vi "ABR-Set Level.vi"(0 "Runtime":T1, 11 "error in (no error)":errorcluster) -> (4 "Runtime out":T1, 14 "Level":dbl, 15 "error out":errorcluster)   [LabVIEW 2020]
uses:
  TypeDefs/ABR-Runtime Data.ctl
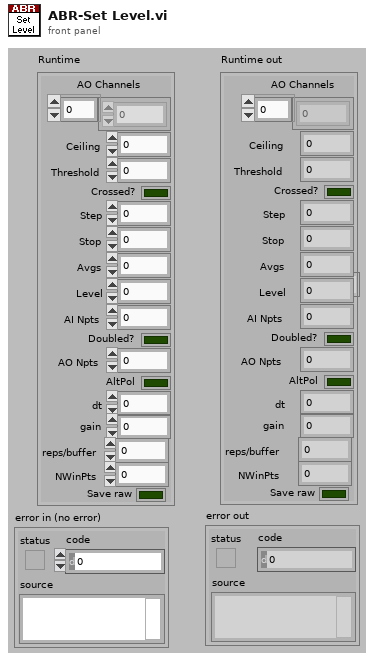
[diagram p1: front panel]
types:
  T1 = typedef "ABR-Runtime Data.ctl" = cluster{"AO Channels":i32[], "Ceiling":dbl, "Threshold":dbl, "Crossed?":bool, "Step":dbl, "Stop":i32, "Avgs":i32, "Level":dbl, "AI Npts":i32, "Doubled?":bool, "AO Npts":i32, "AltPol":bool, "dt":dbl, "gain":dbl, "reps/buffer":i32, "NWinPts":i32, "Save raw":bool}
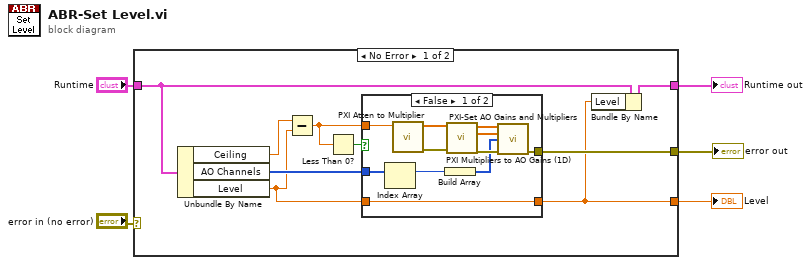
[diagram p0: block diagram]
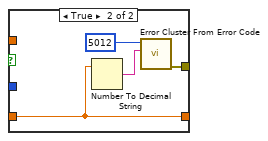
[diagram p2: hidden frame]
diagram:
  n1 = case shown="No Error" "error in (no error)" {
    selector: "error in (no error)" -> [_ w30]
    tunnel: "Runtime" -> [w11 w31]
    tunnel: [w7 w31] -> w3
    tunnel: [w12 w30] -> w2
    tunnel: [w6 _] -> w1
    frame No Error {
      n2 = Unbundle By Name(w11) -> ("Ceiling"=w14:dbl, "AO Channels"=w13:i32[], "Level"=w8:dbl)
      n3 = Subtract(x=w14, y=w8) -> (x-y=w10:dbl)
      n4 = Less Than 0?(x=w10) -> (x < 0?=w9:bool)
      n5 = case shown="False" w9 {
        tunnel: w10 -> [w25 _]
        tunnel: w13 -> [w19 _]
        tunnel: [w17 w29] -> w12
        tunnel: w8 -> [w16 w26]
        tunnel: [w16 w26] -> w6
        frame False {
          n6 = Index Array(array=w19) -> (element=w15:i32)  [unwired: 1 in]
          n7 = call "PXI Atten to Multiplier.vi"("Attenuation"=w25) -> ("error out"=w23:errorcluster, "Multiplier setting"=w24:dbl[])  [unwired: 9 in]
          n8 = Build Array(w15) -> (w18:i32[])
          n9 = call "PXI Multipliers to AO Gains (1D).vi"("Multipliers in"=w24, "error in (no error)"=w23) -> ("Multipliers out"=w20:dbl[], "Gains"=w21:dbl[], "error out"=w22:errorcluster)  [unwired: 11 in]
          n10 = call "PXI-Set AO Gains and Multipliers.vi"("Multipliers"=w20, "Gains"=w21, "AO Channels"=w18, "error in (no error)"=w22) -> ("error out"=w17:errorcluster)  [unwired: 11 in]
        }
        frame True {
          n11 = Number To Decimal String(number=w26) -> (decimal integer string=w27:string)  [unwired: 1 in]
          n12 = call <vilib>:"Error Cluster From Error Code.vi"("error message (\"\")"=w27, "error code (0)"=5012) -> ("error out"=w29:errorcluster)  [unwired: 7 in]
        }
      }
      n13 = Bundle By Name(cluster=w11, "Level"=w6) -> (w7:T1)
    }
    frame Error {
    }
  }
  "error out" <- w2
  "Level" <- w1
  "Runtime out" <- w3
